vi "get_unit_conversion_by_name.vi"(8 "error in (no error)":errorcluster caption="错误输入（无错误）", 10 "name":string, 11 "MotorSystem输入":refnum<class "MotorSystem.lvclass">) -> (0 "error out":errorcluster caption="错误输出", 2 "unit conversion":dbl, 3 "MotorSystem输出":refnum<class "MotorSystem.lvclass">)   [LabVIEW 2016, in "MotionControl_UFO_3DOF.lvlib" / "MotorSystem.lvclass"]
uses:
  <userlib>/MotionControl_UFO_3DOF/MotorSystem/MotorSystem.lvclass
  <userlib>/MotionControl_UFO_3DOF/MotorSystem/MotorSystem.lvclass/MotorSystem.ctl
  <userlib>/MotionControl_UFO_3DOF/OneMotion/OneMotion.lvclass
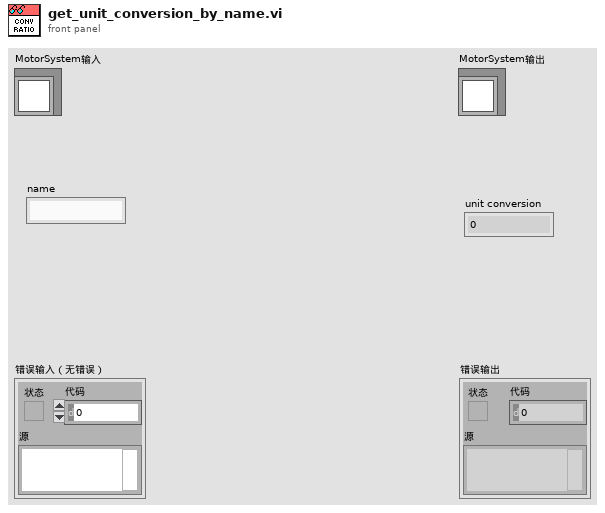
[diagram p1: front panel]
types:
  T1 = typedef "MotionControl_UFO_3DOF.lvlib/MotorSystem.lvclass/MotionCluster.ctl" = cluster{"OneMotion.lvclass":refnum<class "OneMotion.lvclass">, "connected?":bool, "default enabled?":bool, "enabled?":bool}
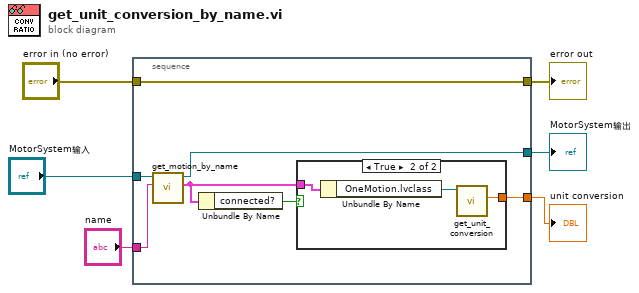
[diagram p0: block diagram]
diagram:
  n1 = stacked-sequence {
    tunnel: [w13] -> w6
    tunnel: [w7] -> w4
    tunnel: "MotorSystem输入" -> [w11]
    tunnel: "error in (no error)" -> [w13]
    tunnel: [w12] -> w1
    tunnel: "name" -> [w10]
    frame #0 {
      n2 = call <userlib>:"get_motion_by_name.vi"("name"=w10, "MotorSystem in"=w11) -> ("motion cluster"=w8:T1, "MotorSystem out"=w7:refnum<class "MotorSystem.lvclass">)  [unwired: 7 in, 1 out]
      n3 = Unbundle By Name(w8) -> ("connected?"=w9:bool)
      n4 = case shown="True" w9 {
        tunnel: w8 -> [_ w16]
        tunnel: [_ w14] -> w12
        frame False {
        }
        frame True {
          n5 = Unbundle By Name(w16) -> ("OneMotion.lvclass"=w15:refnum<class "OneMotion.lvclass">)
          n6 = call-dynamic "get_unit_conversion.vi"("OneMotion输入"=w15) -> ("unit conversion"=w14:dbl)  [unwired: 8 in, 2 out]
        }
      }
    }
  }
  "error out" <- w6
  "MotorSystem输出" <- w4
  "unit conversion" <- w1
